vi "OP600_DCIR.vi"(8 "errin":errorcluster, 9 "Current":dbl, 10 "Durée":sgl, 11 "VISA HITECH":string) -> (0 "errout":errorcluster, 2 "RDCIR":dbl, 3 "Fini?":bool)   [LabVIEW 2020]
uses:
  c2f24cea-a0ab-46e6-be6f-0beeffedb7be.vi
  VG/VG_progressBar.vi
  Carrousel/VarGLO/Global PEAK.vi
  <instrlib>/IT6000C/IT6000C.lvlib
panel:
  out "Actual Current Level (A)":dbl format="%.2g"
  out "Actual Voltage Level (V)":dbl format="%.2g"
  in  "stop":bool
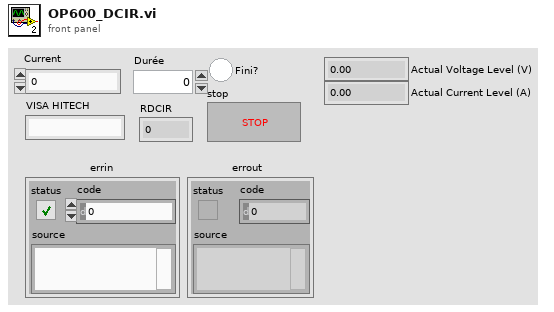
[diagram p1: front panel]
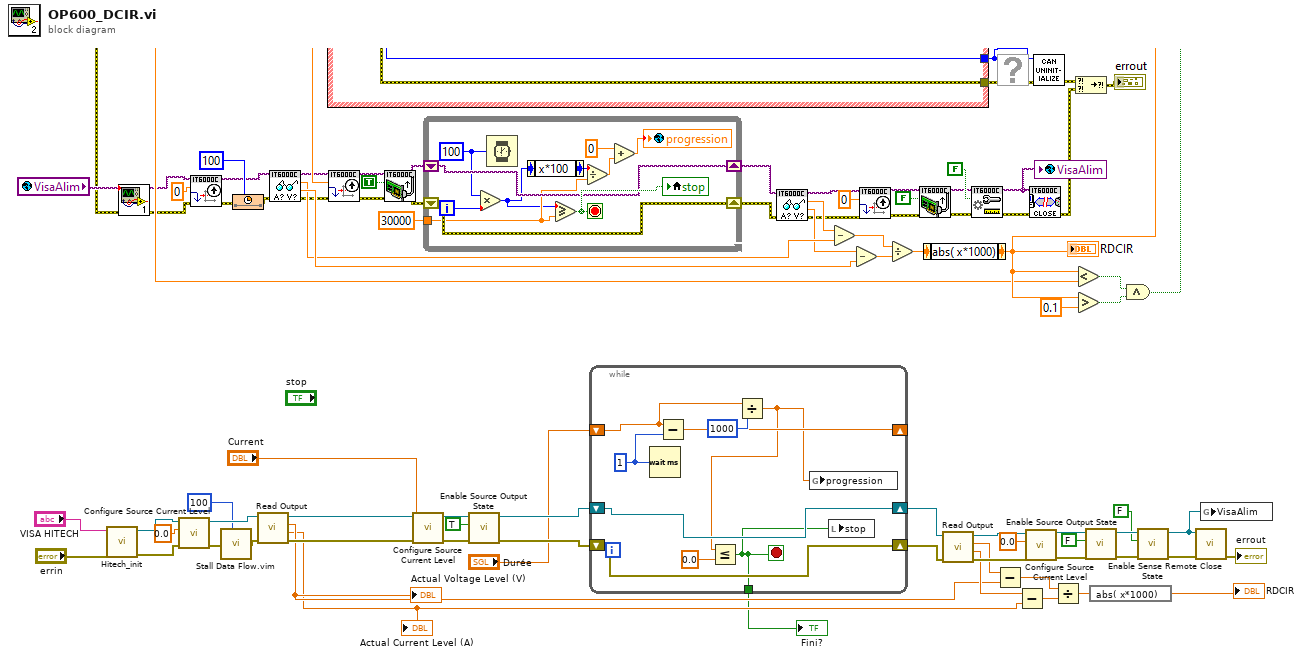
[diagram p0: block diagram]
diagram:
  n1 = call "Hitech_init.vi"("errin"="errin", "VISA HITECH"="VISA HITECH") -> ("error out"=w14:errorcluster, "VisaHitech"=w13:refnum<visa-resource-name>)  [unwired: 8 in]
  n2 = call <instrlib>:"Configure Source Current Level.vi"("error in (no error)"=w14, "Value(0)"=0.0, "VISA resource name"=w13) -> ("error out"=w17:errorcluster, "VISA resource name out"=w40:refnum<visa-resource-name>)  [unwired: 7 in]
  n3 = call "Stall Data Flow.vim"("value in"=w17, "milliseconds to wait"=u32 100) -> ("value out"=w16:errorcluster)  [unwired: 1 out]
  n4 = call <instrlib>:"Read Output.vi"("error in (no error)"=w16, "VISA resource name"=w40) -> ("error out"=w39:errorcluster, "Actual Current Level (A)"=w18:dbl, "Actual Voltage Level (V)"=w19:dbl, "VISA resource name out"=w38:refnum<visa-resource-name>)  [unwired: 6 in]
  "Actual Voltage Level (V)" <- w19
  "Actual Current Level (A)" <- w18
  n5 = call <instrlib>:"Configure Source Current Level.vi"("error in (no error)"=w39, "Value(0)"="Current", "VISA resource name"=w38) -> ("error out"=w37:errorcluster, "VISA resource name out"=w36:refnum<visa-resource-name>)  [unwired: 7 in]
  n6 = call <instrlib>:"Enable Source Output State.vi"("error in (no error)"=w37, "Enable(True)"=TRUE, "VISA resource name"=w36) -> ("error out"=w33:errorcluster, "VISA resource name out"=w34:refnum<visa-resource-name>)  [unwired: 7 in]
  n7 = while {
    shift-right: [w49] -> w20
    shift-left: w34 -> [w49]
    shift-right: [w50] -> w21
    shift-left: w33 -> [w50]
    tunnel: [w44] -> w2
    shift-right: [w45] -> _
    shift-left: "Durée" -> [w47]
    stop <- w44 stop-if-true
    w48 = u32 1 ("attente (ms)")
    n8 = Wait (ms)(milliseconds to wait=w48) -> ()  [unwired: 1 out]
    n9 = Subtract(x=w47, y=w48) -> (x-y=w45:sgl)
    n10 = Divide(x=w47, y=u32 1000) -> (x/y=w43:sgl)
    n11 = Less Or Equal?(x=w43, y=sgl 0.0) -> (x <= y?=w44:bool)
    n12 = global write "VG_progressBar.vi" "progression"(w43) -> ()
    n13 = local write "stop"(w44) -> ()
  }
  "Fini?" <- w2
  n14 = call <instrlib>:"Read Output.vi"("error in (no error)"=w21, "VISA resource name"=w20) -> ("error out"=w31:errorcluster, "Actual Current Level (A)"=w23:dbl, "Actual Voltage Level (V)"=w24:dbl, "VISA resource name out"=w30:refnum<visa-resource-name>)  [unwired: 6 in]
  n15 = Subtract(x=w24, y=w19) -> (x-y=w22:dbl)
  n16 = Subtract(x=w23, y=w18) -> (x-y=w26:dbl)
  n17 = call <instrlib>:"Configure Source Current Level.vi"("error in (no error)"=w31, "Value(0)"=0.0, "VISA resource name"=w30) -> ("error out"=w29:errorcluster, "VISA resource name out"=w28:refnum<visa-resource-name>)  [unwired: 7 in]
  n18 = Divide(x=w22, y=w26) -> (x/y=w25:dbl)
  n19 = call <instrlib>:"Enable Source Output State.vi"("error in (no error)"=w29, "Enable(True)"=FALSE, "VISA resource name"=w28) -> ("error out"=w9:errorcluster, "VISA resource name out"=w11:refnum<visa-resource-name>)  [unwired: 7 in]
  n20 = expression code="abs( x*1000)"(w25) -> (→"RDCIR":dbl)
  n21 = call <instrlib>:"Enable Sense Remote State.vi"("error in (no error)"=w9, "Enable(True)"=FALSE, "VISA resource name"=w11) -> ("error out"=w8:errorcluster, "VISA resource name out"=w10:refnum<visa-resource-name>)  [unwired: 7 in]
  n22 = call <instrlib>:"Close.vi"("error in (no error)"=w8, "VISA resource name"=w10) -> ("error out"=→"errout":errorcluster)  [unwired: 9 in]
  n23 = global write "Global PEAK.vi" "VisaAlim"(w10) -> ()
